vi "间接法谱估计.vi"   [LabVIEW 2018]
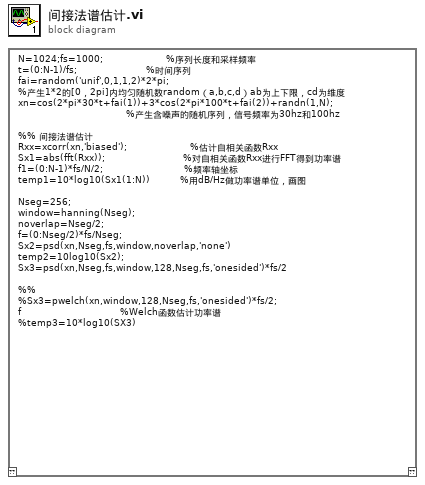
[diagram p0: block diagram]
diagram:
  n1 = mathscript code="N=1024;fs=1000;                     %序列长度和采样频率\nt=(0:N-1)/fs;                       %时间序列\nfai=random('unif',0,1,1,2)*2*pi;    %产生1*2的[0，2pi]内均匀随机数random（a,b,c,d）ab为上下限，cd为维度\nxn=cos(2*pi*30*t+fai(1))+3*cos(2*pi*100*t+fai(2))+randn(1,N);\n                                    %产生含噪声的随机序列，信号频率为30hz和100hz\n\n%% 间接法谱估计\nRxx=xcorr(xn,'biased');                     %估计自相关函数Rxx\nSx1=abs(fft(Rxx));                          %对自相关函数Rxx进行FFT得到功率谱\nf1=(0:N-1)*fs/N/2;                           %频率轴坐标\ntemp1=10*log10(Sx1(1:N))          %用dB/Hz做功率谱单位，画图\n\nNseg=256;\nwindow=hanning(Nseg);\nnoverlap=Nseg/2;\nf=(0:Nseg/2)*fs/Nseg;\nSx2=psd(xn,Nseg,fs,window,noverlap,'none')\ntemp2=10log10(Sx2);\nSx3=psd(xn,Nseg,fs,window,128,Nseg,fs,'onesided')*fs/2\n\n%% \n%Sx3=pwelch(xn,window,128,Nseg,fs,'onesided')*fs/2;\nf                                 %Welch函数估计功率谱\n%temp3=10*log10(SX3)"() -> ()  [unwired: 1 in, 1 out]
